vi "Stepper SM Step.vi"(8 "Step Count in":i32, 10 "Half period (ticks)":i16=10000, 11 "Edges (2)":i32=2) -> (0 "Step Count out":i32)   [LabVIEW 2015]
uses:
  <vilib>/rvi/eio/common/nirviEmuTemplateMethod_errors.vi
  <vilib>/eio/EIONode/EIONode.xnode
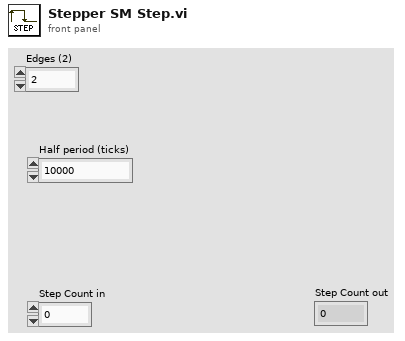
[diagram p1: front panel]
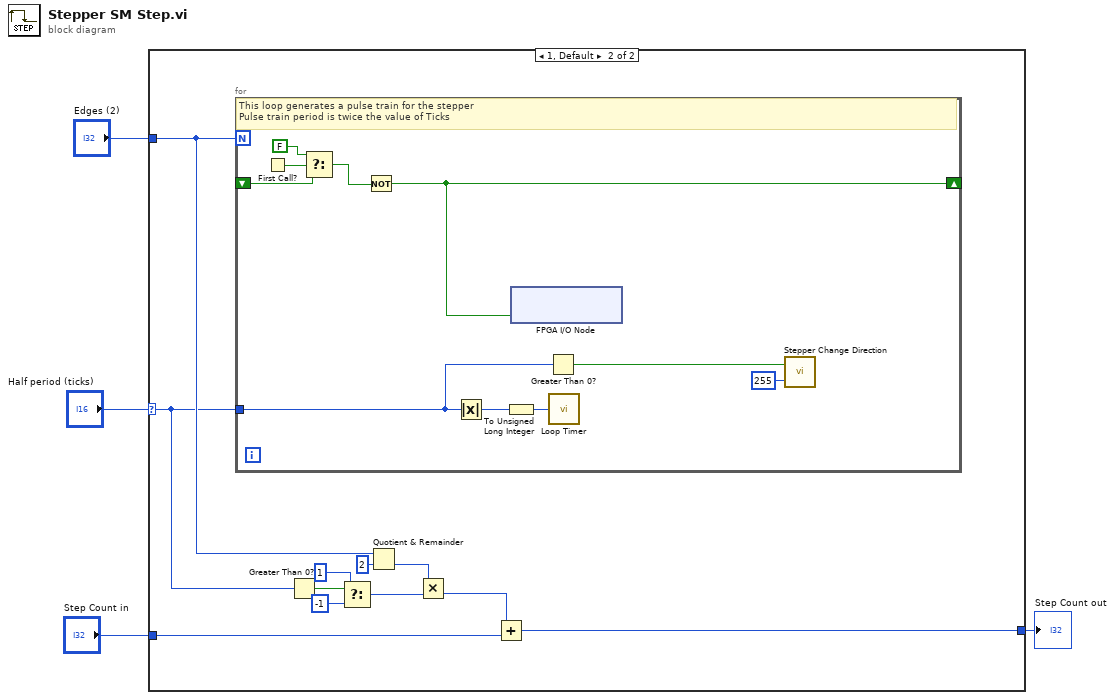
[diagram p0: block diagram]
diagram:
  n1 = case shown="1, Default" "Half period (ticks)" {
    selector: "Half period (ticks)" -> [_ w6]
    tunnel: "Step Count in" -> [w5 w13]
    tunnel: [w5 w11] -> w2
    tunnel: "Edges (2)" -> [_ w9]
    frame 0 {
    }
    frame 1, Default {
      n2 = for {
        N: w9 -> [_]
        shift-right: [w24] -> _
        shift-left: _ -> [w21]
        tunnel: w6 -> [w17]
        # "This loop generates a pulse train for the stepper\nPulse train period is twice the value of Ticks"
        n3 = First Call?() -> (First Call?: T/F=w23:bool)
        n4 = Select(t=FALSE, s=w23, f=w21) -> (s? t:f=w20:bool)
        n5 = Not(x=w20) -> (.not. x?=w24:bool)
        n6 = Absolute Value(x=w17) -> (abs(x)=w25:i16)
        n7 = To Unsigned Long Integer(number=w25) -> (unsigned 32bit integer=w26:u32)
        n8 = xnode "FPGA I/O Node"("Stepper/Step"=w24) -> ()  [unwired: 1 in, 1 out]
        n9 = Greater Than 0?(x=w17) -> (x > 0?=w19:bool)
        n10 = call "Loop Timer"("Count(Ticks)"=w26) -> ()  [unwired: 1 out]
        n11 = call "Stepper Change Direction.vi"("Wait before changing (Ticks)"=u8 255, "Direction (T=Home)"=w19) -> ()  [unwired: 2 in]
      }
      n12 = Greater Than 0?(x=w6) -> (x > 0?=w16:bool)
      n13 = Select(t=1, s=w16, f=-1) -> (s? t:f=w12:i32)
      n14 = Quotient & Remainder(x=w9, y=2) -> (floor(x/y)=w7:i32)  [unwired: 1 out]
      n15 = Multiply(x=w7, y=w12) -> (x*y=w10:i32)
      n16 = Add(x=w10, y=w13) -> (x+y=w11:i32)
    }
  }
  "Step Count out" <- w2
